vi "Processing_HistProperties.vi"(0 "Histogram":i32[][](array[numeric]), 1 "Minimum Piezo (-0.25) / nm":dbl=-0.25, 3 "Maximum Piezo (3.2) / nm":dbl=3.2, 11 "2D intensity":dbl(slide)=5.1020408163265305 scale=0.0..50.0, 12 "Minimum Log(G/G0) (-6)":dbl=-6.0, 13 "Maximum Log(G/G0) (0.5)":dbl=0.5) -> (4 "Intensity Graph Input":dbl[][](array[numeric]), 6 "2DHist-ZScale.MarkerVals[]":cluster{sgl, u32}[](array[cluster]), 8 "2DHist-YScale.Ofst&Mult":cluster{"Minimum Log(G/G0)":dbl, dbl}, 10 "2DHist-XScale.Ofst&Mult":cluster{"Minimum Log(G/G0)":dbl, dbl}, 14 "1DHist-XScale.Ofst&Mult":cluster{"Minimum Log(G/G0)":dbl, dbl}, 15 "2DHist-ZScale.HighColor":u32(colorbox)=10756619)   [LabVIEW 2023]
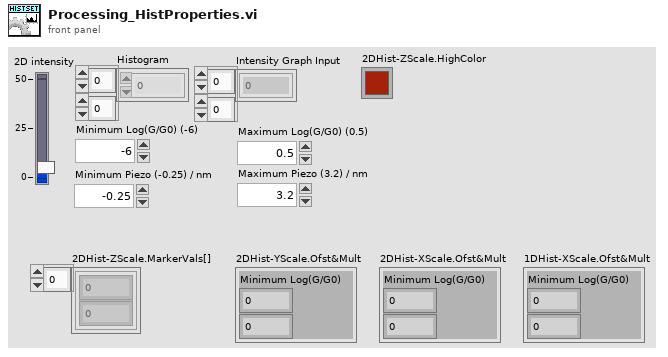
[diagram p1: front panel]
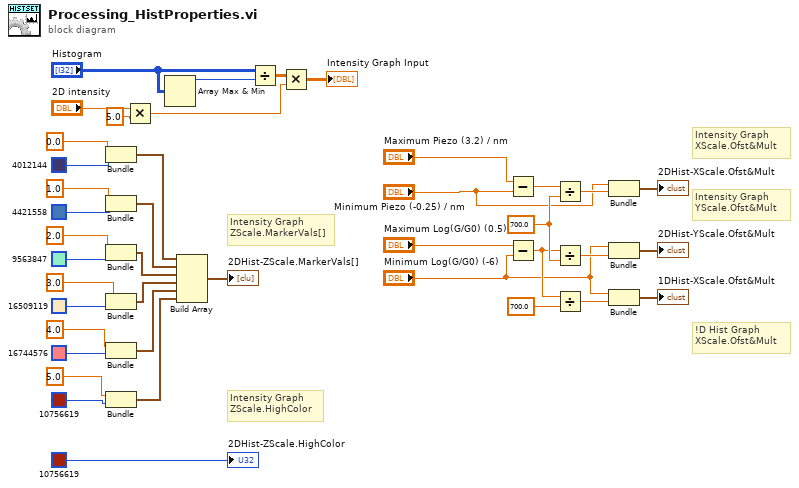
[diagram p0: block diagram]
diagram:
  w13 = 700.0 ("y")
  # "Intensity Graph\nZScale.HighColor"
  # "!D Hist Graph\nXScale.Ofst&Mult"
  # "Intensity Graph\nXScale.Ofst&Mult"
  # "Intensity Graph\nYScale.Ofst&Mult"
  # "Intensity Graph\nZScale.MarkerVals[]"
  n1 = Bundle(sgl 0.0, u32 4012144) -> (w34:cluster{sgl, u32})  [unwired: 1 in]
  n2 = Bundle(sgl 1.0, u32 4421558) -> (w33:cluster{sgl, u32})  [unwired: 1 in]
  n3 = Bundle(sgl 2.0, u32 9563847) -> (w32:cluster{sgl, u32})  [unwired: 1 in]
  n4 = Bundle(sgl 3.0, u32 16509119) -> (w31:cluster{sgl, u32})  [unwired: 1 in]
  n5 = Bundle(sgl 4.0, u32 16744576) -> (w30:cluster{sgl, u32})  [unwired: 1 in]
  n6 = Bundle(sgl 5.0, u32 10756619) -> (w29:cluster{sgl, u32})  [unwired: 1 in]
  n7 = Multiply(x="2D intensity", y=5.0) -> (x*y=w37:dbl)
  n8 = Array Max & Min(array="Histogram") -> (max value=w41:i32)  [unwired: 3 out]
  n9 = Build Array(w34, w33, w32, w31, w30, w29) -> (→"2DHist-ZScale.MarkerVals[]":cluster{sgl, u32}[])
  n10 = Divide(x="Histogram", y=w41) -> (x/y=w40:dbl[][])
  n11 = Multiply(x=w40, y=w37) -> (x*y=→"Intensity Graph Input":dbl[][])
  n12 = Subtract(x="Maximum Piezo (3.2) / nm", y="Minimum Piezo (-0.25) / nm") -> (x-y=w14:dbl)
  n13 = Subtract(x="Maximum Log(G/G0) (0.5)", y="Minimum Log(G/G0) (-6)") -> (x-y=w9:dbl)
  n14 = Divide(x=w14, y=w13) -> (x/y=w11:dbl)
  n15 = Divide(x=w9, y=w13) -> (x/y=w12:dbl)
  n16 = Divide(x=w9, y=700.0) -> (x/y=w7:dbl)
  n17 = Bundle("Minimum Piezo (-0.25) / nm"="Minimum Piezo (-0.25) / nm", w11) -> (→"2DHist-XScale.Ofst&Mult":cluster{"Minimum Piezo (-0.25) / nm":dbl, dbl})  [unwired: 1 in]
  n18 = Bundle("Minimum Log(G/G0) (-6)"="Minimum Log(G/G0) (-6)", w12) -> (→"2DHist-YScale.Ofst&Mult":cluster{"Minimum Log(G/G0) (-6)":dbl, dbl})  [unwired: 1 in]
  n19 = Bundle("Minimum Log(G/G0) (-6)"="Minimum Log(G/G0) (-6)", w7) -> (→"1DHist-XScale.Ofst&Mult":cluster{"Minimum Log(G/G0) (-6)":dbl, dbl})  [unwired: 1 in]
  "2DHist-ZScale.HighColor" <- u32 10756619
